vi "AlliGator Harmonic Orders String.vi"(2 "Harmonic Order Array":u8[](array[numeric])) -> (7 "String":string)   [LabVIEW 2021, in "AlliGator Files.lvlib"]
doc: "Creates harmonic order string ."
uses:
  AlliGator Files.lvlib
panel:
  # "see the AlliGator License on the block diagram (Ctrl+E or Window:Show Block Diagram)"
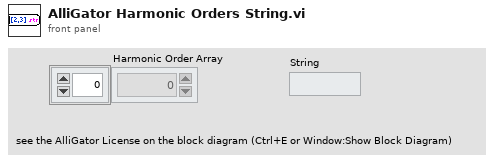
[diagram p1: front panel]
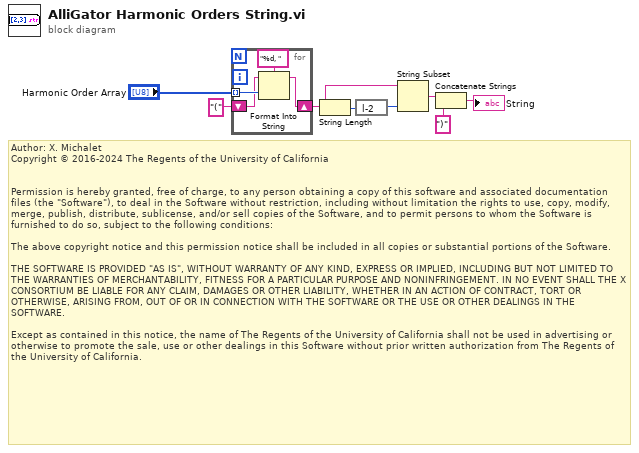
[diagram p0: block diagram]
diagram:
  # "Author: X. Michalet\nCopyright © 2016-2024 The Regents of the University of California\n \n\nPermission is hereby granted, free of charge, to any person obtaining a copy of this software and associated documentation files (the \"Software\"), to deal in the Software without restriction, including without limitation the rights to use, copy, modify, merge, publish, distribute, sublicense, and/or sell copies of the Software, and to permit persons to whom the Software is furnished to do so, subject to the following conditions:\n\nThe above copyright notice and this permission notice shall be included in all copies or substantial portions of the Software.\n\nTHE SOFTWARE IS PROVIDED \"AS IS\", WITHOUT WARRANTY OF ANY KIND, EXPRESS OR IMPLIED, INCLUDING BUT NOT LIMITED TO THE WARRANTIES OF MERCHANTABILITY, FITNESS FOR A PARTICULAR PURPOSE AND NONINFRINGEMENT. IN NO EVENT SHALL THE X CONSORTIUM BE LIABLE FOR ANY CLAIM, DAMAGES OR OTHER LIABILITY, WHETHER IN AN ACTION OF CONTRACT, TORT OR OTHERWISE, ARISING FROM, OUT OF OR IN CONNECTION WITH THE SOFTWARE OR THE USE OR OTHER DEALINGS IN THE SOFTWARE.\n\nExcept as contained in this notice, the name of The Regents of the University of California shall not be used in advertising or otherwise to promote the sale, use or other dealings in this Software without prior written authorization from The Regents of the University of California."
  n1 = for {
    tunnel: "Harmonic Order Array" -> [w12] mode=indexing
    shift-right: [w9] -> w5
    shift-left: "(" -> [w11]
    n2 = Format Into String(format string="%d, ", initial string=w11, w12) -> (resulting string=w9:string)  [unwired: 1 in, 1 out]
  }
  n3 = String Length(string=w5) -> (length=w8:i32)
  n4 = expression code="l-2"(w8) -> (w4:i32)
  n5 = String Subset(string=w5, length (rest)=w4) -> (substring=w3:string)  [unwired: 1 in]
  n6 = Concatenate Strings(w3, ")" ("string")) -> (→"String":string)
